vi "Relative position conversion.vi"(11 "Position":T1) -> (3 "position abs":cluster{"Left":i32, "Top":i32})   [LabVIEW 2023]
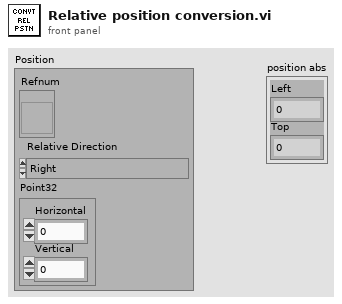
[diagram p1: front panel]
types:
  T1 = cluster{"Refnum":refnum<vi>, "Relative Direction":enum32{"Right", "Left", "Top", "Bottom", "Top Right", "Top Left", "Bottom Right", "Bottom Left"}, "Point32":cluster{"Horizontal":i32, "Vertical":i32}}
  T2 = typedef "LVPositionTypeDef.ctl" = cluster{"Left":i32, "Top":i32}
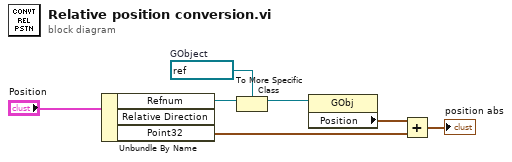
[diagram p0: block diagram]
diagram:
  w4 = refnum<vi> refnum  # GObject
  n1 = Unbundle By Name("Position") -> ("Refnum"=w6:refnum<vi>, "Point32"=w2:cluster{"Horizontal":i32, "Vertical":i32})  [unwired: 1 out]
  n2 = To More Specific Class(target class=w4, reference=w6) -> (specific class reference=w5:refnum<vi>)  [unwired: 1 in, 1 out]
  n3 = property class="GObj"(reference=w5) -> ("Position"=w3:T2)  [unwired: 1 in, 2 out]
  n4 = Add(x=w3, y=w2) -> (x+y=→"position abs":T2)
